vi "Queue Comms Get Elements.vi"(8 "error in (no error)":errorcluster) -> (0 "error out":errorcluster, 2 "elements":T1[](array[typedef]))   [LabVIEW 2014, in "Controller (Host).lvlib"]
doc: "This subVI dequeues an element from the communications queue using the Queue Comms FGV"
uses:
  Controller (Host).lvlib
  Private Controls/Module Data.ctl
  Private Controls/Module Action.ctl
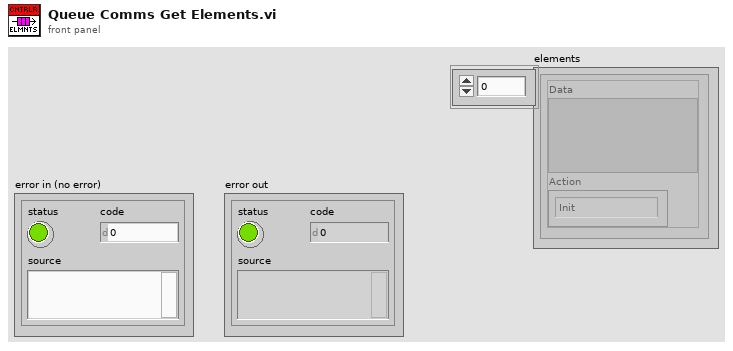
[diagram p1: front panel]
types:
  T1 = typedef "Controller (Host).lvlib/Module Data.ctl" = cluster{"Data":variant, "Action":T2}
  T2 = typedef "Controller (Host).lvlib/Module Action.ctl" = enum8{"Timeout", "Init", "Error", "Exit", "Set cRIO Connected Status", "Prompt Login", "Prompt Main Menu", "Prompt APU Select", "Prompt Operation Select", "Prompt SubTests Select", "Prompt Break Out", "Calibration", "Testing", "Load User Info", "Set Instr Init Status", "Load APU Setup Data", "Engine Start Val Change", "RPM Cross 95Perc Thresh", "Interactive Ctrls Val Change"}
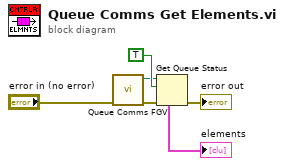
[diagram p0: block diagram]
diagram:
  n1 = call "Queue Comms FGV.vi"("error in (no error)"="error in (no error)") -> ("error out"=w2:errorcluster, "Queue out"=w3:refnum<queue>)  [unwired: 9 in]
  n2 = Get Queue Status(queue=w3, return elements? (F)=TRUE, error in (no error)=w2) -> (error out=→"error out":errorcluster, elements=→"elements":T1[])  [unwired: 6 out]
